vi "OpenSensor.vi"(0 "Fehler (Eingang, kein Fehler)":errorcluster, 5 "instanceHandle":u32, 7 "DLL-Path":path, 11 "COM_Port":string) -> (4 "Fehler (Ausgang)":errorcluster, 6 "instanceHandle":u32, 8 "DLL-Path":path, 10 "ERR_CODE":i32)   [LabVIEW 2015, in "MEDAQLib.lvlib"]
doc: "ERR_CODE OpenSensor (DWORD instanceHandle);\n\nEstablish the connection to the sensor. After connecting to the sensor,\nall internal parameters starting with SP_, CP_ and IP_ are cleared (like at\nfunction ClearAllParameters)."
uses:
  MEDAQLib.lvlib
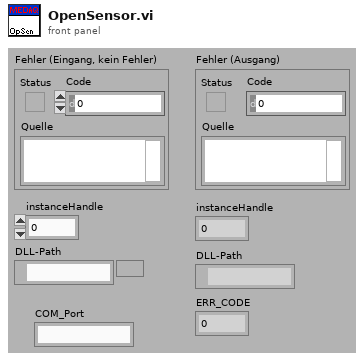
[diagram p1: front panel]
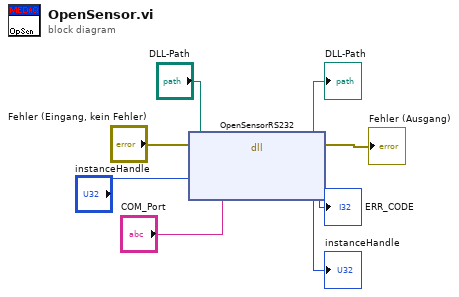
[diagram p0: block diagram]
diagram:
  n1 = dll-call lib="C:/Programme/National Instruments 8.6/LabVIEW 8.6/instr.lib/MEDAQLib/Release/MEDAQLib.dll" fn="OpenSensorRS232"(path in="DLL-Path", error in="Fehler (Eingang, kein Fehler)", "instanceHandle"="instanceHandle", "COM_Port"="COM_Port") -> (path out=→"DLL-Path":path, error out=→"Fehler (Ausgang)":errorcluster, "Rückgabetyp"=→"ERR_CODE":i32, "instanceHandle"=→"instanceHandle":u32)  [unwired: 2 in]
